vi "getExptFolder.vi"(8 "error in (no error)":errorcluster, 11 "Inst.Transport in":refnum<class "Inst.Transport.lvclass">) -> (0 "error out":errorcluster, 2 "folder":string, 3 "Inst.Transport out":refnum<class "Inst.Transport.lvclass">)   [LabVIEW 2019, in "Inst.Transport.lvclass"]
uses:
  Inst.Transport.lvclass
  Typedefs/Inst.Transport.PublicCommands--Enum.ctl
  Typedefs/ExptFolder--RequestResponse--Cluster.ctl
  3e889260-abcf-4491-902b-eb5ea8ef53e4.vi
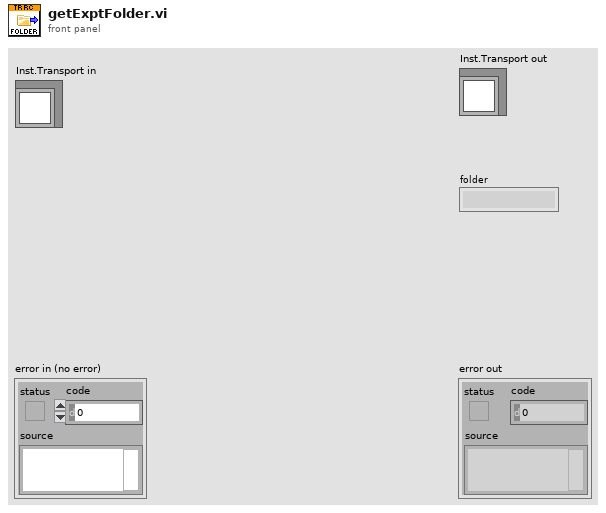
[diagram p1: front panel]
types:
  T1 = typedef "Inst.Transport.lvclass/ExptFolder--RequestResponse--Cluster.ctl" = cluster{"folder":string}
  T2 = typedef "Inst.Transport.lvclass/Inst.Transport.PublicCommands--Enum.ctl" = enum16{"startTransport", "stopTransport", "getStatus", "setExptFolder", "getExptFolder", "setExptComments", "getExptComments", "setExptParam", "appendExptParam", "clearExptParam", "setSweepConfig", "getSweepConfig"}
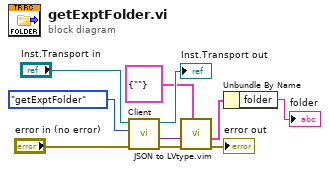
[diagram p0: block diagram]
diagram:
  n1 = call-dynamic "Client.vi"("error in (no error)"="error in (no error)", "Command in"=Inst.Transport.PublicCommands--Enum."getExptFolder" ("Commands"), "Instrument in"="Inst.Transport in") -> ("error out"=w2:errorcluster, "Data out"=w3:variant, "Instrument out"=→"Inst.Transport out":refnum<class "Inst.Transport.lvclass">)  [unwired: 5 in, 1 out]
  n2 = call "JSON to LVtype.vim"("type"=T1 {"folder"=""} ("setExptFolder"), "error in (no error)"=w2, "JSON Data in"=w3) -> ("error out"=→"error out":errorcluster, "Data out"=w5:T1)  [unwired: 7 in]
  n3 = Unbundle By Name(w5) -> ("folder"=→"folder":string)
